vi "Read switch_state.vi"(8 "error in (no error)":errorcluster, 11 "Z_HSw in":refnum<class "Z_HSw.lvclass">) -> (0 "error out":errorcluster, 2 "button state":T1, 3 "Z_HSw out":refnum<class "Z_HSw.lvclass">)   [LabVIEW 2019, in "Z_HSw.lvclass"]
uses:
  Z_HSw.lvclass
  ctl/Z_HSw_state.ctl
  Z_HSw.lvclass/Z_HSw.ctl
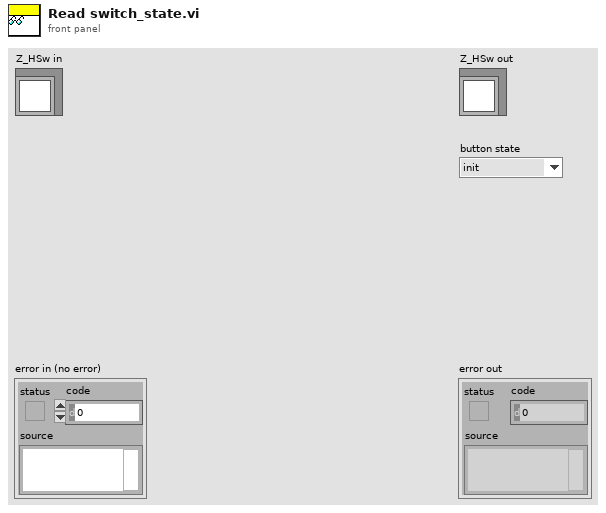
[diagram p1: front panel]
types:
  T1 = typedef "Z_HSw.lvclass/Z_HSw_state.ctl" = enum16{"init", "switch hand", "not hand", "hand", "switch auto", "not auto", "auto"}
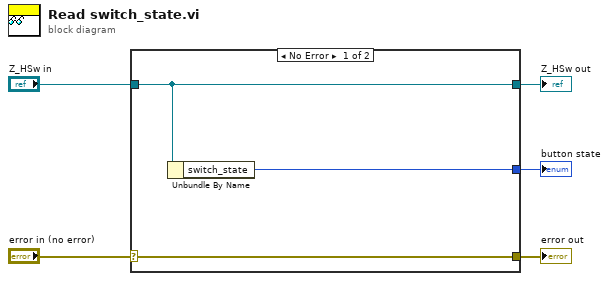
[diagram p0: block diagram]
diagram:
  n1 = case shown="No Error" "error in (no error)" {
    selector: "error in (no error)" -> [w8 w9]
    tunnel: [w8 w9] -> w4
    tunnel: [w7 w10] -> w2
    tunnel: "Z_HSw in" -> [w7 w10]
    tunnel: [w6 _] -> w1
    frame No Error {
      n2 = Unbundle By Name(w7) -> ("switch_state"=w6:T1)
    }
    frame Error {
    }
  }
  "error out" <- w4
  "Z_HSw out" <- w2
  "button state" <- w1
